vi "lab8.vi"() -> ()   [LabVIEW 2020]
uses:
  <vilib>/measure/NI_MABase.lvlib
  <vilib>/measure/NI_MAPro.lvlib
  <vilib>/gmath/NI_Gmath.lvlib
  <vilib>/Analysis/NI_AALPro.lvlib
  <vilib>/Analysis/2dsp.llb/Power Spectrum (DBL).vi
  <vilib>/measure/macond.llb/IIR Filter for 1 Chan.vi
  <vilib>/Analysis/4window.llb/Hamming Window (DBL).vi
  <vilib>/Analysis/4window.llb/Blackman Window (DBL).vi
  <vilib>/Analysis/4window.llb/Blackman-Harris Window (DBL).vi
  <vilib>/Analysis/4window.llb/Cosine Tapered Window (DBL).vi
  <vilib>/Analysis/3filter.llb/Filter Structure Type.ctl
  <vilib>/Analysis/NI_AALBase.lvlib
panel:
  in  "Modulation sig type":T1(ring)
  out "Modulation settings":enum32{"AM", "PM", "FM"}(tab)
  in  "M":dbl
  in  "Modulation type":enum16{"AM", "PM", "FM"}(ring)
  in  "?":bool
  in  "signal type":T1(ring)
  in  "Frequncy":dbl
  in  "Phase":dbl
  in  "Amplitude 3":dbl
  in  "Square duty cycle, %":dbl
  in  "Offset":dbl
  in  "Reset":bool
  in  "Mean":dbl
  in  "Order":dbl
  in  "Start freq":dbl
  in  "Delta freq":dbl
  in  "Amplitude 2":dbl
  in  "noise type":T2(ring)
  in  "Reset Noise":bool
  in  "Filter specifications":T3={"Topology"=enum."Butterworth", "Type"=enum."Lowpass", "Order"=1, "Lower Fc"=100.0, "Upper Fc"=200.0, "PB Ripple"=1.0, "SB Attenuation"=60.0} {"PB Ripple" format="%0.2f"; "SB Attenuation" format="%0.2f"; "Lower Fc" format="%0.2p"; "Upper Fc" format="%0.2p"}
  in  "filter structure option":T4=10 items=["IIR 2nd Order"=0, "IIR 4th Order"=1, "Auto Select"=10]
  in  "Window type":T5(ring)
  in  "?":T6(tab)
  out "?":sgl[][](graph)
  out "Filtered Spectrum":dbl[](graph)
  out "Windowed Spectrum":dbl[](graph)
  out "Signal":waveform(dbl)(graph)
  out "Noise":waveform(dbl)(graph)
  out "Sig + noise":waveform(dbl)(graph)
  out "Filtered":waveform(dbl)(graph)
  in  "Amplitude":dbl=1.0 format="%.2p"
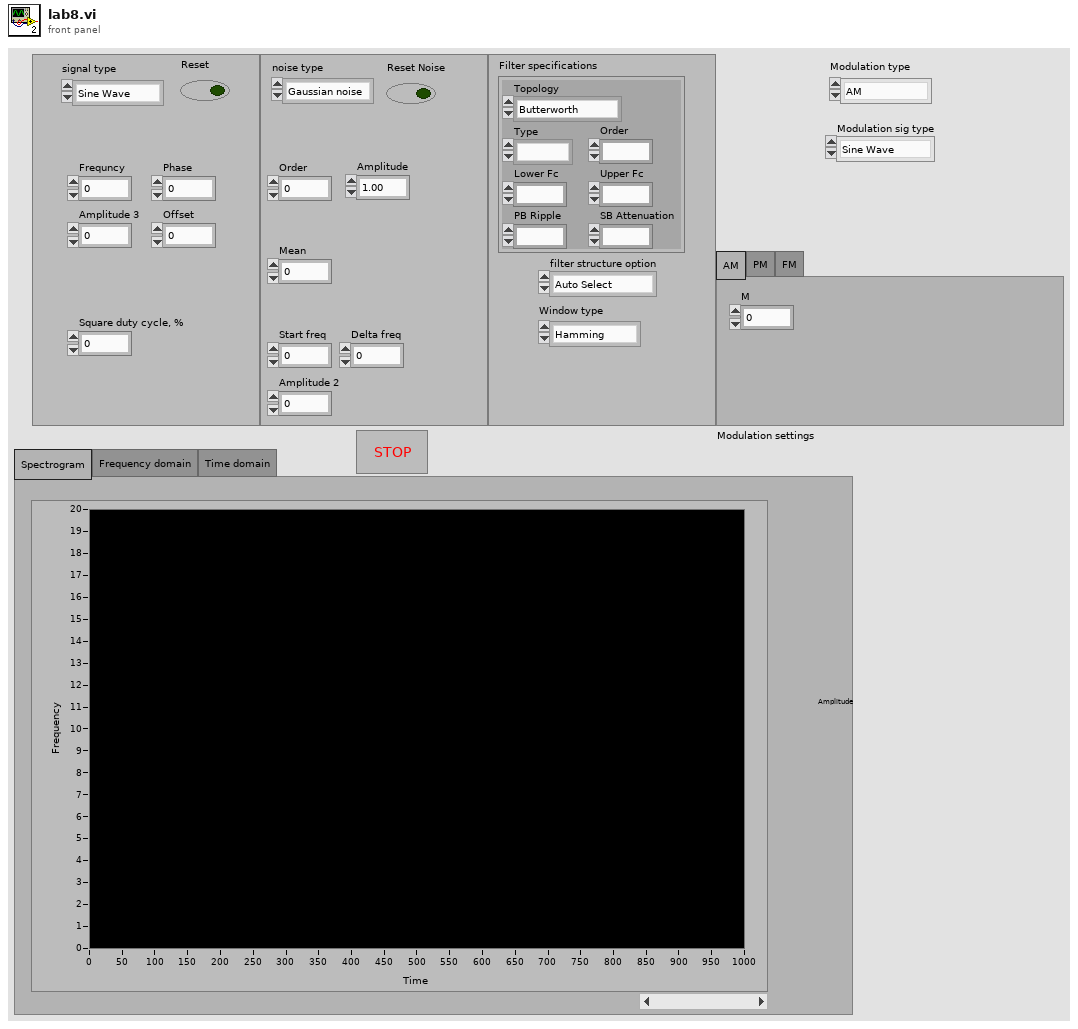
[diagram p1: front panel]
types:
  T1 = enum16{"Sine Wave", "Triangle Wave", "Square Wave", "Sawtooth Wave"}
  T2 = enum16{"Gaussian noise", "Multitone Noise", "Gamma Noise", "Poisson Noise"}
  T3 = cluster{"Topology":enum16{"Off", "Butterworth", "Chebyshev", "Inverse Chebyshev", "Elliptic", "Bessel"}, "Type":enum16{"Lowpass", "Highpass", "Bandpass", "Bandstop"}, "Order":i32, "Lower Fc":dbl, "Upper Fc":dbl, "PB Ripple":dbl, "SB Attenuation":dbl}
  T4 = typedef "NI_AALBase.lvlib/Filter Structure Type.ctl" = u16
  T5 = enum16{"Hamming", "Blackman", "Blackman-Harris", "Tapered cos"}
  T6 = enum32{"Spectrogram", "Frequency domain", "Time domain"}
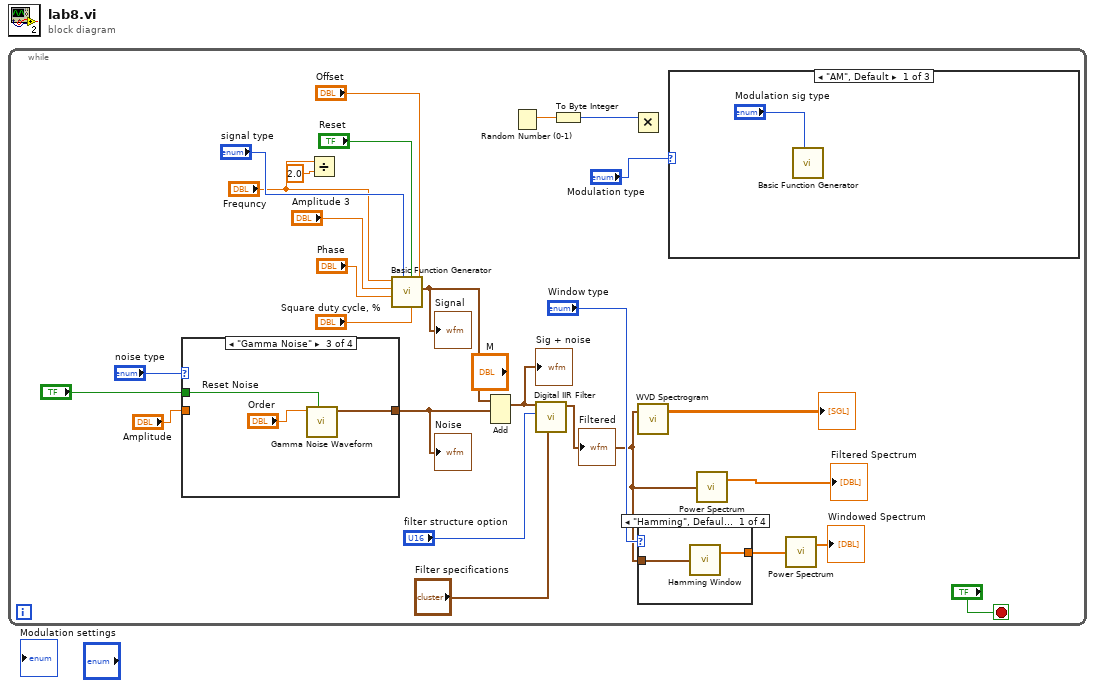
[diagram p0: block diagram]
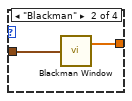
[diagram p4: hidden frame]
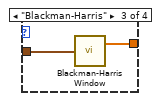
[diagram p5: hidden frame]
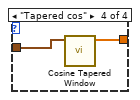
[diagram p6: hidden frame]
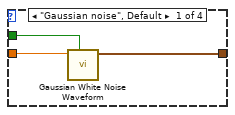
[diagram p7: hidden frame]
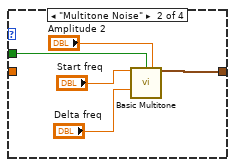
[diagram p8: hidden frame]
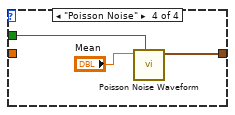
[diagram p9: hidden frame]
diagram:
  n1 = while {
    stop <- "?" stop-if-true
    n2 = case shown="\"Gamma Noise\"" "noise type" {
      tunnel: [w38 w42 w45 w47] -> w15
      tunnel: "Reset Noise" -> [w37 w43 w44 w49]
      tunnel: "Amplitude" -> [w36 _ _ _]
      frame "Gaussian noise", Default {
        n3 = call <vilib>:"Gaussian White Noise Waveform.vi"("reset signal"=w37, "standard deviation"=w36) -> ("signal out"=w38:waveform(dbl))  [unwired: 8 in, 1 out]
      }
      frame "Multitone Noise" {
        n4 = call <vilib>:"Basic Multitone.vi"("start frequency"="Start freq", "reset signal"=w43, "amplitude"="Amplitude 2", "delta frequency"="Delta freq") -> ("signal out"=w42:waveform(dbl))  [unwired: 8 in, 3 out]
      }
      frame "Gamma Noise" {
        n5 = call <vilib>:"Gamma Noise Waveform.vi"("reset signal"=w44, "order"="Order") -> ("signal out"=w45:waveform(dbl))  [unwired: 8 in, 1 out]
      }
      frame "Poisson Noise" {
        n6 = call <vilib>:"Poisson Noise Waveform.vi"("reset signal"=w49, "mean"="Mean") -> ("signal out"=w47:waveform(dbl))  [unwired: 8 in, 1 out]
      }
    }
    "Noise" <- w15
    n7 = Divide(x="Frequncy", y=2.0) -> ()  [unwired: 1 out]
    n8 = call <vilib>:"Basic Function Generator.vi"("offset"="Offset", "square wave duty cycle (%)"="Square duty cycle, %", "reset signal"="Reset", "signal type"="signal type", "phase"="Phase", "amplitude"="Amplitude 3", "frequency"="Frequncy") -> ("signal out"=w4:waveform(dbl))  [unwired: 2 in, 2 out]
    "Signal" <- w4
    n9 = Add(1:w15, 2:w4) -> (0:w6:waveform(dbl))  [unwired: 1 in, 1 out]
    "Sig + noise" <- w6
    n10 = Random Number (0-1)() -> (number: 0 to 1=w3:dbl)
    n11 = call-poly <vilib>:"Digital IIR Filter.vi"("IIR filter specifications"="Filter specifications", "filter structure option"="filter structure option", "signal in"=w6) -> ("signal out"=w9:waveform(dbl))  [unwired: 6 in, 2 out]
    "Filtered" <- w9
    n12 = To Byte Integer(number=w3) -> (8bit integer=w2:i8)
    n13 = Multiply(x=w2) -> ()  [unwired: 1 in, 1 out]
    n14 = call <vilib>:"WVD Spectrogram.vi"("X"=w9) -> ("WVD Spectrogram {X}"=→"?":sgl[][])  [unwired: 1 in, 1 out]
    n15 = case shown="\"Hamming\", Default" "Window type" {
      tunnel: w9 -> [w29 w31 w33 w35]
      tunnel: [w28 w30 w32 w34] -> w8
      frame "Hamming", Default {
        n16 = call-poly <vilib>:"Hamming Window.vi"("X"=w29) -> ("Windowed X"=w28:dbl[])  [unwired: 1 out]
      }
      frame "Blackman" {
        n17 = call-poly <vilib>:"Blackman Window.vi"("X"=w31) -> ("Windowed X"=w30:dbl[])  [unwired: 1 out]
      }
      frame "Blackman-Harris" {
        n18 = call-poly <vilib>:"Blackman-Harris Window.vi"("X"=w33) -> ("Windowed X"=w32:dbl[])  [unwired: 1 out]
      }
      frame "Tapered cos" {
        n19 = call-poly <vilib>:"Cosine Tapered Window.vi"("X"=w35) -> ("Windowed X"=w34:dbl[])  [unwired: 9 in, 1 out]
      }
    }
    n20 = case shown="\"AM\", Default" "Modulation type" {
      frame "AM", Default {
        n21 = call <vilib>:"Basic Function Generator.vi"("signal type"="Modulation sig type") -> ()  [unwired: 8 in, 3 out]
      }
      frame "PM" {
      }
      frame "FM" {
      }
    }
    n22 = call-poly <vilib>:"Power Spectrum.vi"("X"=w9) -> ("Power Spectrum"=→"Filtered Spectrum":dbl[])  [unwired: 1 out]
    n23 = call-poly <vilib>:"Power Spectrum.vi"("X"=w8) -> ("Power Spectrum"=→"Windowed Spectrum":dbl[])  [unwired: 1 out]
  }
